vi "Check File Log Thresholds.vi"(8 "log thresholds":T2 {"Segment Files By" items=["Time", "Size"]}, 9 "Hard Drive Space Used (%)":dbl, 11 "Log file Size MB":dbl) -> (2 "Elapsed Time (s)":dbl, 3 "action":T1(ring))   [LabVIEW 2020, in "Frame Logging.lvlib"]
uses:
  Frame Logging.lvlib
  Shared/loggingThreshold_types.ctl
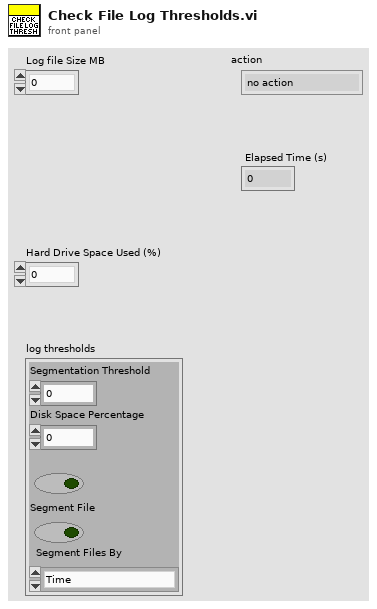
[diagram p1: front panel]
types:
  T1 = enum16{"no action", "close file", "segment file"}
  T2 = typedef "loggingThreshold_types.ctl" = cluster{"Segmentation Threshold":dbl, "Disk Space Percentage":dbl, "Check Disk Space":bool, "Segment File":bool, "Segment Files By":u16}
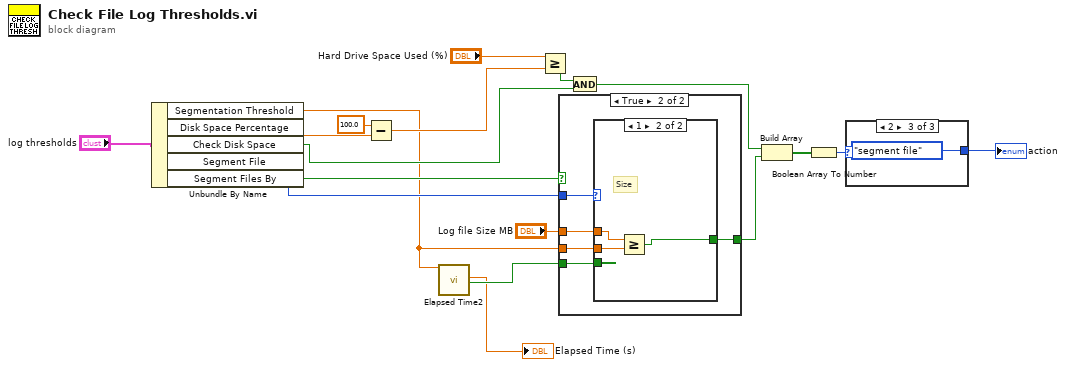
[diagram p0: block diagram]
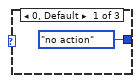
[diagram p2: hidden frame]
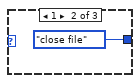
[diagram p3: hidden frame]
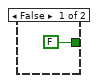
[diagram p4: hidden frame]
diagram:
  n1 = Unbundle By Name("log thresholds") -> ("Segmentation Threshold"=w2:dbl, "Disk Space Percentage"=w9:dbl, "Check Disk Space"=w8:bool, "Segment File"=w7:bool, "Segment Files By"=w6:u16)
  n2 = Subtract(x=100.0 ("y"), y=w9) -> (x-y=w5:dbl)
  n3 = call "Elapsed Time2"("Time Target (s)"=w2) -> ("Elapsed Time (s)"=→"Elapsed Time (s)":dbl, "Time has Elapsed"=w3:bool)  [unwired: 11 in, 6 out]
  n4 = Greater Or Equal?(x="Hard Drive Space Used (%)", y=w5) -> (x >= y?=w16:bool)
  n5 = case shown="True" w7 {
    tunnel: w6 -> [_ w24]
    tunnel: "Log file Size MB" -> [_ w21]
    tunnel: [FALSE w23] -> w13
    tunnel: w3 -> [_ w22]
    tunnel: w2 -> [_ w20]
    frame False {
    }
    frame True {
      n6 = case shown="1" w24 {
        tunnel: w22 -> [w25 _]
        tunnel: [w25 w26] -> w23
        tunnel: w21 -> [_ w28]
        tunnel: w20 -> [_ w27]
        frame 0, Default {
          # "Time"
        }
        frame 1 {
          # "Size"
          n7 = Greater Or Equal?(x=w28, y=w27) -> (x >= y?=w26:bool)
        }
      }
    }
  }
  n8 = And(x=w16, y=w8) -> (x .and. y?=w14:bool)
  n9 = Build Array(w14, w13) -> (w12:bool[])
  n10 = Boolean Array To Number(Boolean array=w12) -> (number=w11:u32)
  n11 = case shown="2" w11 {
    tunnel: [T1."no action" ("action") T1."close file" ("action") T1."segment file" ("action")] -> w10
    frame 0, Default {
    }
    frame 1 {
    }
    frame 2 {
    }
  }
  "action" <- w10
